vi "Actor Core.vi"(8 "error in":errorcluster, 11 "Plant in":refnum<class "Plant.lvclass">) -> (0 "error out":errorcluster, 3 "Actor out":refnum<class "Actor.lvclass">)   [LabVIEW 2023, in "Plant.lvlib" / "Plant.lvclass"]
doc: "(<B>Filename</B>: Actor Framework.lvlib:Actor.lvclass:Actor Core.vi)\n\nReceives messages to the actor, reacts to them, and initiates any error handling that may shut the actor down.\n\nDescendant classes may override this VI to append parallel tasks for the actor to complete while it handles messages. Overrides use the Call Parent Class Method node."
uses:
  Plant.lvclass
  Plant.lvclass/Plant.ctl
  Plant Messages/Run Step Msg/Run Step Msg.lvclass
  <vilib>/ActorFramework/Message Enqueuer/Message Enqueuer.lvclass
  <vilib>/ActorFramework/Actor/Actor.lvclass
  C:/Program Files (x86)/National Instruments/LabVIEW 2023/vi.lib/ActorFramework/Actor/Actor.lvclass
  C:/Projects/RESTws/Examples/Actor Framework/Plant/Plant/Plant.lvclass
  GUI/GUI.lvclass
  C:/Projects/RESTws/Examples/Actor Framework/GUI/GUI.lvclass
  C:/Program Files (x86)/National Instruments/LabVIEW 2023/vi.lib/ActorFramework/Message/Message.lvclass
  C:/Projects/RESTws/Examples/Actor Framework/Plant/Plant Messages/Run Step Msg/Run Step Msg.lvclass
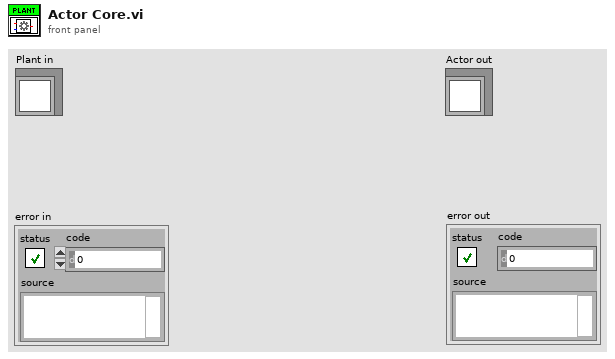
[diagram p1: front panel]
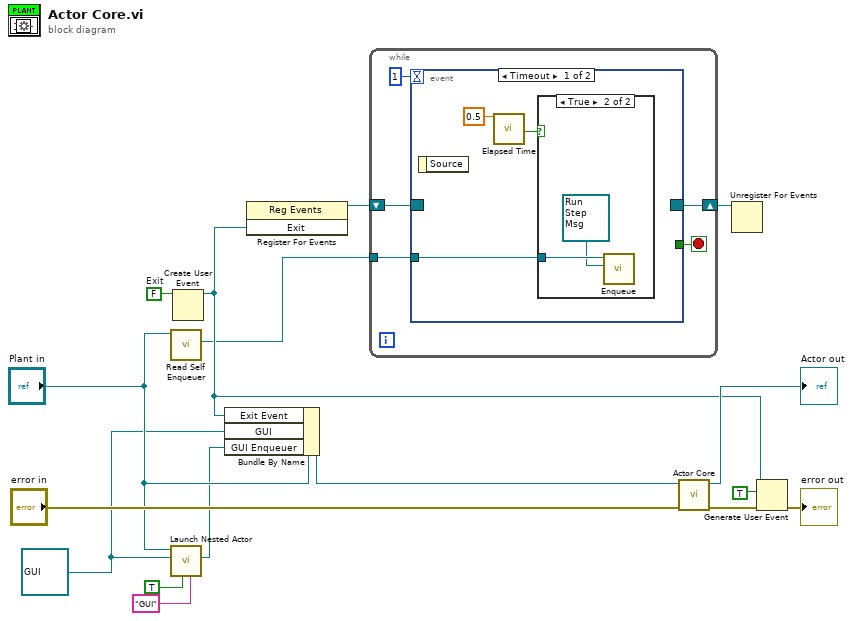
[diagram p0: block diagram]
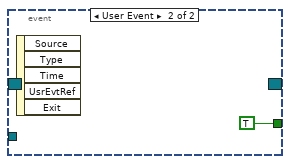
[diagram p3: hidden frame]
diagram:
  w6 = refnum<class "GUI.lvclass"> refnum ("GUI.lvlib:GUI.lvclass")
  w2 = FALSE  # Exit
  n1 = call <vilib>:"Read Self Enqueuer.vi"("Actor"="Plant in") -> ("Self Enqueuer"=w8:refnum<class "Message Enqueuer.lvclass">)  [unwired: 10 in]
  n2 = call <vilib>:"Launch Nested Actor.vi"("Debug Alias"="GUI", "Open Actor Core front panel? (F)"=TRUE, "Nested Actor"=w6, "Caller Actor in"="Plant in") -> ("Nested Actor's Enqueuer"=w5:refnum<class "Message Enqueuer.lvclass">)  [unwired: 5 in, 2 out]
  n3 = Create User Event(user event datatype=w2) -> (user event=w10:refnum<user-event>)  [unwired: 1 in, 1 out]
  n4 = Bundle By Name(cluster="Plant in", "Exit Event"=w10, "GUI"=w6, "GUI Enqueuer"=w5) -> (w13:refnum<class "Plant.lvclass">)
  n5 = register-events(w10) -> (reference out=w14:refnum<event-registration>)  [unwired: 2 in, 1 out]
  n6 = while {
    tunnel: w8 -> [w19]
    shift-right: [w17] -> w1
    shift-left: w14 -> [w21]
    stop <- w18 stop-if-true
    n7 = event shown="[0] Timeout" {
      selector: w21 -> [_ _]
      dyn-events: [_ _] -> w17
      timeout: 1 -> [_ _]
      tunnel: w19 -> [w22 _]
      tunnel: [_ TRUE] -> w18
      event Timeout {
        n8 = event-data() -> ()  [unwired: 1 in, 1 out]
        n9 = call "Elapsed Time"("Time Target (s)"=0.5) -> ("Time has Elapsed"=w23:bool)  [unwired: 11 in, 7 out]
        n10 = case shown="True" w23 {
          tunnel: w22 -> [_ w26]
          frame False {
          }
          frame True {
            n11 = call <vilib>:"Enqueue.vi"("Message"=refnum<class "Run Step Msg.lvclass"> refnum ("Plant.lvlib:Run Step Msg.lvclass"), "Message Enqueuer in"=w26) -> ()  [unwired: 8 in, 2 out]
          }
        }
      }
      event User Event {
        n12 = event-data() -> ()  [unwired: 1 in, 5 out]
      }
    }
  }
  n13 = call-parent "Actor Core.vi"("error in"="error in", "Actor in"=w13) -> ("error out"=w12:errorcluster, "Actor out"=→"Actor out":refnum<class "Actor.lvclass">)  [unwired: 8 in]
  n14 = Unregister For Events(event registration refnum=w1) -> ()  [unwired: 1 in, 1 out]
  n15 = Generate User Event(user event=w10, event data cluster=TRUE, error in=w12) -> (error out=→"error out":errorcluster)  [unwired: 1 in, 1 out]
